vi "conexion_internet.vi"() -> (2 "Internet status":string="No Internet connection", 3 "Internet connection":bool)   [LabVIEW 2015]
uses:
  <vilib>/httpClient/LabVIEWHTTPClient.lvlib
panel:
  out "standard output":string
  out "error out":errorcluster
  in  "error in (no error)":errorcluster
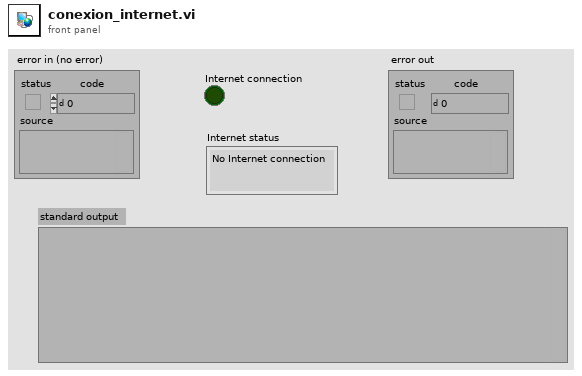
[diagram p1: front panel]
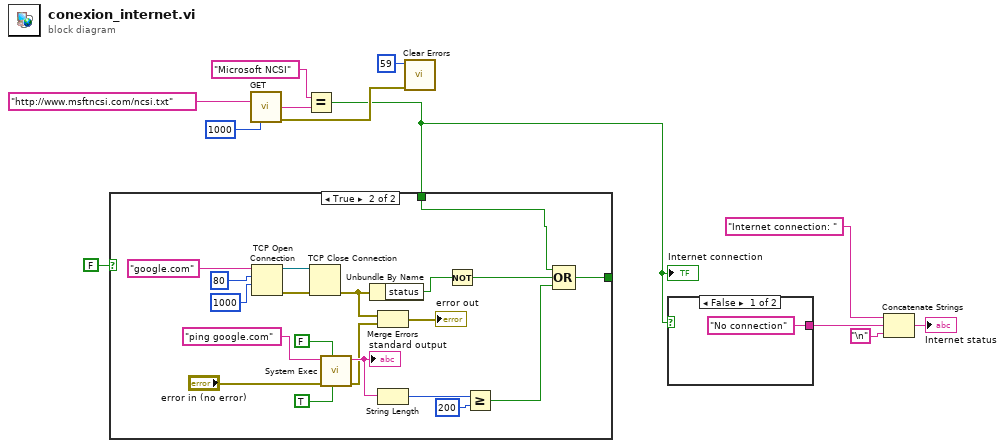
[diagram p0: block diagram]
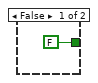
[diagram p2: hidden frame]
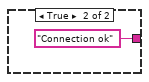
[diagram p3: hidden frame]
diagram:
  n1 = call <vilib>:"GET.vi"("url"="http://www.msftncsi.com/ncsi.txt", "timeout (10000)"=1000) -> ("body"=w5:string, "error out"=w4:errorcluster)  [unwired: 10 in, 2 out]
  n2 = Equal?(x="Microsoft NCSI", y=w5) -> (x = y?=w3:bool)
  "Internet connection" <- w3
  n3 = case shown="True" FALSE {
    tunnel: [FALSE w15] -> _
    tunnel: w3 -> [_ w14]
    frame False {
    }
    frame True {
      n4 = TCP Open Connection(address="google.com", remote port or service name=u16 80, timeout ms (60000)=1000) -> (connection ID=w26:refnum<k5>, error out=w27:errorcluster)  [unwired: 2 in]
      n5 = TCP Close Connection(connection ID=w26, error in (no error)=w27) -> (error out=w21:errorcluster)  [unwired: 1 in, 1 out]
      n6 = call <vilib>:"System Exec.vi"("run minimized? (F)"=TRUE, "wait until completion? (T)"=FALSE, "error in (no error)"="error in (no error)", "command line"="ping google.com") -> ("error out"=w22:errorcluster, "standard output"=w31:string)  [unwired: 4 in, 2 out]
      "standard output" <- w31
      n7 = Unbundle By Name(w21) -> ("status"=w23:bool)
      n8 = Merge Errors(w21, w22) -> (→"error out":errorcluster)
      n9 = String Length(string=w31) -> (length=w30:i32)
      n10 = Not(x=w23) -> (.not. x?=w17:bool)
      n11 = Greater Or Equal?(x=w30, y=200) -> (x >= y?=w16:bool)
      n12 = Compound Arithmetic op=OR(w14, w17, w16) -> (w15:bool)
    }
  }
  n13 = call <vilib>:"Clear Errors.vi"("error in (no error)"=w4, "specific error code to clear (0: all)"=59) -> ()  [unwired: 4 in, 2 out]
  n14 = case shown="False" w3 {
    tunnel: ["No connection" "Connection ok"] -> w12
    frame False {
    }
    frame True {
    }
  }
  n15 = Concatenate Strings("Internet connection: " ("string"), w12, "\n") -> (→"Internet status":string)
